vi "Utility Config File Read_01.vi"(6 "Controls Excluded":refnum<vi>[](array[refnum]), 8 "Error In":errorcluster, 10 "Path":path, 11 "Controls In":refnum<vi>[](array[refnum])) -> (0 "Error Out":errorcluster, 1 "Fixe Exists?":bool, 2 "Values":variant[](array[variant]), 3 "Controls Out":refnum<vi>[](array[refnum]), 4 "Path_Out":path)   [LabVIEW 2020]
uses:
  <vilib>/Utility/config.llb/Read Key (String).vi
  <vilib>/Utility/config.llb/NI_LVConfig.lvlib
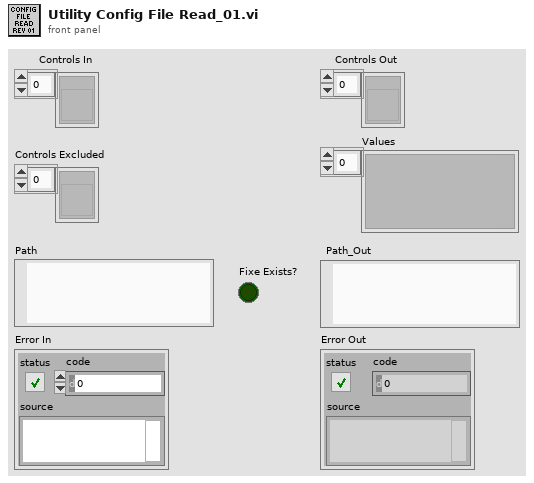
[diagram p1: front panel]
types:
  T1 = typedef "NI_LVConfig.lvlib/Config Data RefNum.ctl" = refnum<k1>
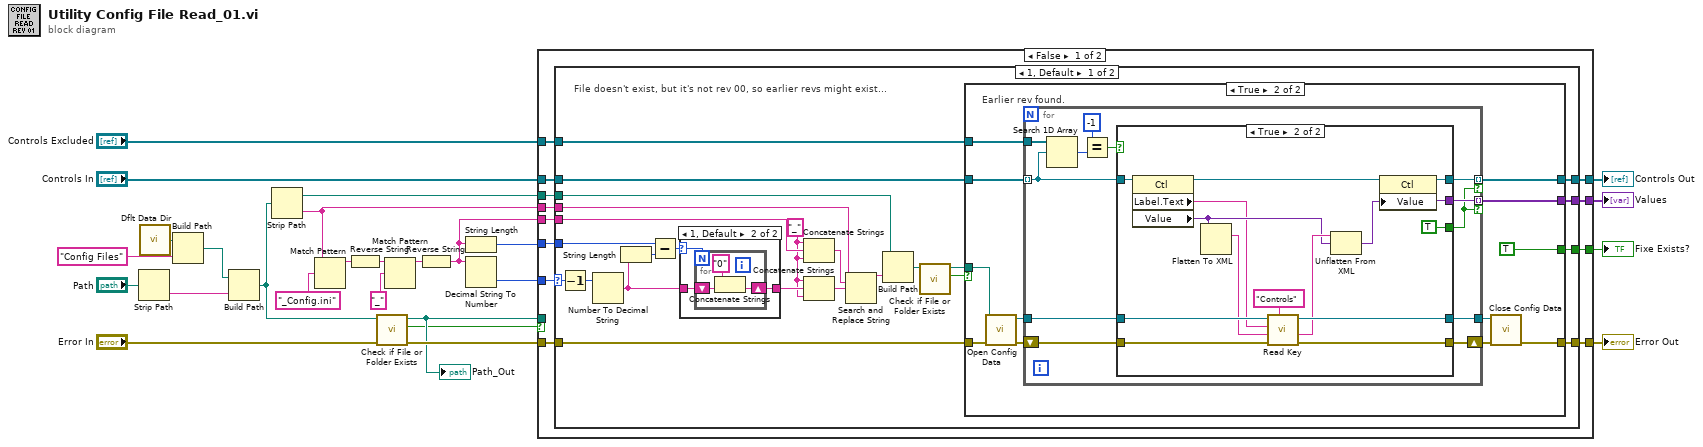
[diagram p0: block diagram]
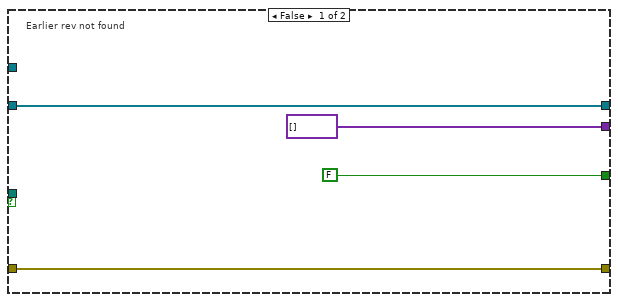
[diagram p2: hidden frame]
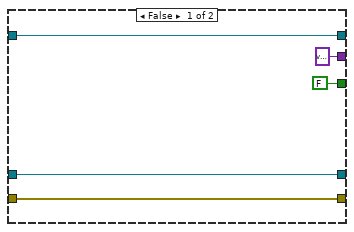
[diagram p3: hidden frame]
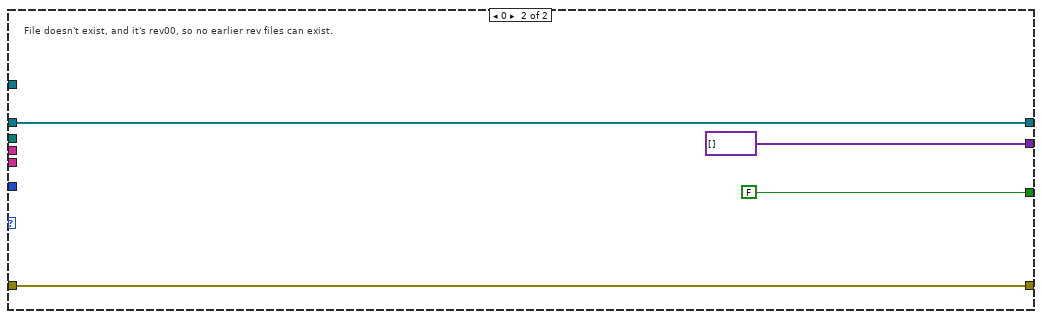
[diagram p5: hidden frame]
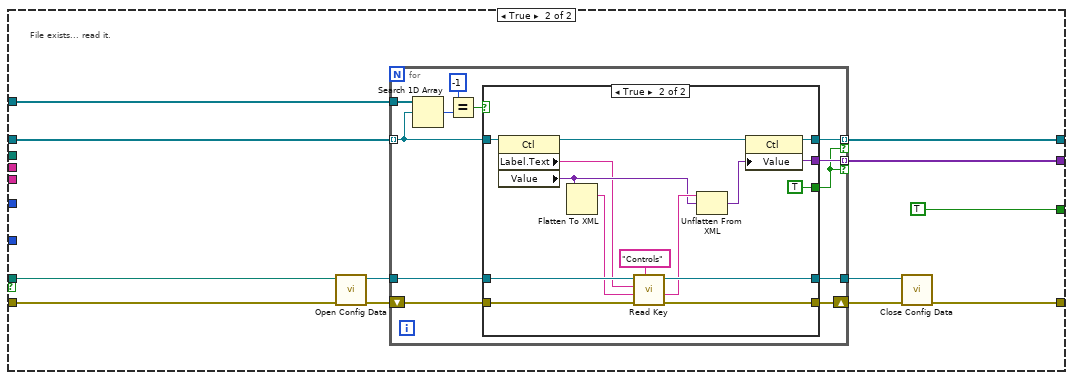
[diagram p6: hidden frame]
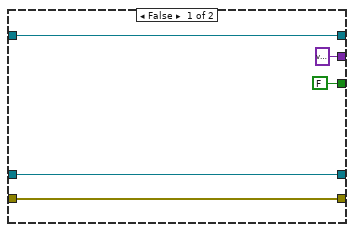
[diagram p7: hidden frame]
diagram:
  n1 = Strip Path(path="Path") -> (name=w1:string)  [unwired: 1 out]
  n2 = call <vilib>:"Dflt Data Dir.vi"() -> ("App:Default Data Directory"=w15:path)
  n3 = Build Path(base path=w15, name or relative path="Config Files") -> (appended path=w13:path)
  n4 = Build Path(base path=w13, name or relative path=w1) -> (appended path=w4:path)
  n5 = Strip Path(path=w4) -> (stripped path=w3:path, name=w7:string)
  n6 = Match Pattern(string=w7, regular expression="_Config.ini") -> (before substring=w11:string)  [unwired: 1 in, 3 out]
  n7 = Reverse String(1:w11) -> (0:w10:string)
  n8 = call <vilib>:"Check if File or Folder Exists.vi"("error in (no error)"="Error In", "path"=w4) -> ("error out"=w22:errorcluster, "file or folder exists?"=w18:bool, "dup path"=w21:path)  [unwired: 7 in]
  "Path_Out" <- w21
  n9 = Match Pattern(string=w10, regular expression="_") -> (before substring=w5:string)  [unwired: 1 in, 3 out]
  n10 = Reverse String(1:w5) -> (0:w2:string)
  n11 = String Length(string=w2) -> (length=w6:i32)
  n12 = Decimal String To Number(string=w2) -> (number=w8:i32)  [unwired: 2 in, 1 out]
  n13 = case shown="False" w18 {
    tunnel: "Controls In" -> [w31 w130]
    tunnel: [w33 w129] -> w24
    tunnel: w22 -> [w34 w128]
    tunnel: w21 -> [_ w127]
    tunnel: [w32 w126] -> w20
    tunnel: [w38 w125] -> w19
    tunnel: [w37 TRUE] -> w17
    tunnel: "Controls Excluded" -> [w30 w123]
    tunnel: w8 -> [w36 _]
    tunnel: w7 -> [w35 _]
    tunnel: w6 -> [w29 _]
    tunnel: w2 -> [w28 _]
    tunnel: w3 -> [w27 _]
    frame False {
      n14 = case shown="1, Default" w36 {
        selector: w36 -> [w56 _]
        tunnel: [w60 variant[] []] -> w38
        tunnel: [w61 FALSE] -> w37
        tunnel: w35 -> [w50 _]
        tunnel: w34 -> [w40 w118]
        tunnel: [w62 w118] -> w33
        tunnel: [w59 w117] -> w32
        tunnel: w31 -> [w58 w117]
        tunnel: w30 -> [w57 _]
        tunnel: w29 -> [w53 _]
        tunnel: w28 -> [w49 _]
        tunnel: w27 -> [w44 _]
        frame 1, Default {
          w47 = "_" ("regular expression")
          # "File doesn't exist, but it's not rev 00, so earlier revs might exist..."
          n15 = Decrement(x=w56) -> (x-1=w55:i32)
          n16 = Number To Decimal String(number=w55) -> (decimal integer string=w54:string)  [unwired: 1 in]
          n17 = String Length(string=w54) -> (length=w52:i32)
          n18 = Subtract(x=w53, y=w52) -> (x-y=w51:i32)
          n19 = case shown="1, Default" w51 {
            selector: w51 -> [_ w111]
            tunnel: w54 -> [w110 w113]
            tunnel: [w110 w112] -> w48
            frame 0 {
            }
            frame 1, Default {
              n20 = for {
                N: w111 -> [_]
                shift-right: [w114] -> w112
                shift-left: w113 -> [w116]
                n21 = Concatenate Strings("0" ("string"), w116) -> (w114:string)
              }
            }
          }
          n22 = Concatenate Strings(w47, w49, w47) -> (w46:string)
          n23 = Concatenate Strings(w47, w48, w47) -> (w45:string)
          n24 = Search and Replace String(input string=w50, search string=w46, replace string=w45) -> (result string=w43:string)  [unwired: 5 in, 3 out]
          n25 = Build Path(base path=w44, name or relative path=w43) -> (appended path=w42:path)
          n26 = call <vilib>:"Check if File or Folder Exists.vi"("path"=w42) -> ("file or folder exists?"=w39:bool, "dup path"=w41:path)  [unwired: 8 in, 1 out]
          n27 = case shown="True" w39 {
            tunnel: [w64 w74] -> w62
            tunnel: [FALSE TRUE] -> w61
            tunnel: [variant[] [] w72] -> w60
            tunnel: [w63 w71] -> w59
            tunnel: w58 -> [w63 w70]
            tunnel: w57 -> [_ w69]
            tunnel: w41 -> [_ w68]
            tunnel: w40 -> [w64 w67]
            frame False {
              # "Earlier rev not found"
            }
            frame True {
              # "Earlier rev found."
              n28 = call <vilib>:"Open Config Data.vi"("error in (no error)"=w67, "configuration file path"=w68) -> ("error out"=w75:errorcluster, "refnum"=w76:T1)  [unwired: 1 in, 7 out]
              n29 = for {
                shift-right: [w88] -> w78
                shift-left: w75 -> [w89]
                tunnel: w70 -> [w81] mode=indexing
                tunnel: [w86] -> w72 mode=indexing if=w79
                tunnel: [w85] -> w71 mode=indexing if=w79
                tunnel: w69 -> [w84]
                tunnel: w76 -> [w90]
                tunnel: [w87] -> w77
                n30 = Search 1D Array(1D array=w84, element=w81) -> (index of element=w83:i32)  [unwired: 1 in]
                n31 = Equal?(x=-1, y=w83) -> (x = y?=w80:bool)
                n32 = case shown="True" w80 {
                  tunnel: w90 -> [w92 w109]
                  tunnel: w89 -> [w91 w108]
                  tunnel: [w91 w106] -> w88
                  tunnel: [w92 w105] -> w87
                  tunnel: [variant ("Value") w100] -> w86
                  tunnel: [w95 w99] -> w85
                  tunnel: w81 -> [w95 w97]
                  tunnel: [FALSE TRUE] -> w79
                  frame False {
                  }
                  frame True {
                    n33 = property class="Ctl"(reference=w97) -> (reference out=w98:refnum<vi>, "Label.Text"=w101:string, "Value"=w102:variant)  [unwired: 1 in, 1 out]
                    n34 = Flatten To XML(6:w102) -> (2:w104:string)
                    n35 = call-poly <vilib>:"Read Key.vi"("section"="Controls", "error in (no error)"=w108, "default value"=w104, "key"=w101, "refnum"=w109) -> ("error out"=w106:errorcluster, "value"=w103:string, "refnum out"=w105:T1)  [unwired: 3 in, 1 out]
                    n36 = Unflatten From XML(xml string=w103, type=w102) -> (value=w100:variant)  [unwired: 1 in, 1 out]
                    n37 = property class="Ctl"(reference=w98, "Value"=w100) -> (reference out=w99:refnum<vi>)  [unwired: 1 in, 1 out]
                  }
                }
              }
              n38 = call <vilib>:"Close Config Data.vi"("error in (no error)"=w78, "refnum"=w77) -> ("error out"=w74:errorcluster)  [unwired: 1 in, 8 out]
            }
          }
        }
        frame 0 {
          # "File doesn't exist, and it's rev00, so no earlier rev files can exist."
        }
      }
    }
    frame True {
      # "File exists... read it."
      n39 = call <vilib>:"Open Config Data.vi"("error in (no error)"=w128, "configuration file path"=w127) -> ("error out"=w121:errorcluster, "refnum"=w122:T1)  [unwired: 1 in, 7 out]
      n40 = for {
        shift-right: [w142] -> w132
        shift-left: w121 -> [w143]
        tunnel: w130 -> [w135] mode=indexing
        tunnel: [w140] -> w125 mode=indexing if=w133
        tunnel: [w139] -> w126 mode=indexing if=w133
        tunnel: w123 -> [w138]
        tunnel: w122 -> [w144]
        tunnel: [w141] -> w131
        n41 = Search 1D Array(1D array=w138, element=w135) -> (index of element=w137:i32)  [unwired: 1 in]
        n42 = Equal?(x=-1, y=w137) -> (x = y?=w134:bool)
        n43 = case shown="True" w134 {
          tunnel: w144 -> [w146 w163]
          tunnel: w143 -> [w145 w162]
          tunnel: [w145 w160] -> w142
          tunnel: [w146 w159] -> w141
          tunnel: [variant ("Value") w154] -> w140
          tunnel: [w149 w153] -> w139
          tunnel: w135 -> [w149 w151]
          tunnel: [FALSE TRUE] -> w133
          frame False {
          }
          frame True {
            n44 = property class="Ctl"(reference=w151) -> (reference out=w152:refnum<vi>, "Label.Text"=w155:string, "Value"=w156:variant)  [unwired: 1 in, 1 out]
            n45 = Flatten To XML(6:w156) -> (2:w158:string)
            n46 = call-poly <vilib>:"Read Key.vi"("section"="Controls", "error in (no error)"=w162, "default value"=w158, "key"=w155, "refnum"=w163) -> ("error out"=w160:errorcluster, "value"=w157:string, "refnum out"=w159:T1)  [unwired: 3 in, 1 out]
            n47 = Unflatten From XML(xml string=w157, type=w156) -> (value=w154:variant)  [unwired: 1 in, 1 out]
            n48 = property class="Ctl"(reference=w152, "Value"=w154) -> (reference out=w153:refnum<vi>)  [unwired: 1 in, 1 out]
          }
        }
      }
      n49 = call <vilib>:"Close Config Data.vi"("error in (no error)"=w132, "refnum"=w131) -> ("error out"=w129:errorcluster)  [unwired: 1 in, 8 out]
    }
  }
  "Error Out" <- w24
  "Controls Out" <- w20
  "Values" <- w19
  "Fixe Exists?" <- w17
